vi "PCI8622模拟量采集.vi"() -> (0 "3通道":dbl, 1 "2通道":dbl, 2 "1通道":dbl, 3 "0通道":dbl)   [LabVIEW 2011]
panel:
  in  "超时时间(秒)":i32 min=0 max=3600
  in  "接地方式":i32(ring) items=["单端方式", "差分方式"]
  in  "触发灵敏窗(25nS)":i32=100 min=1 max=65535
  in  "分组间隔(uS)":i32=100 min=0 max=419430
  in  "采样频率(Hz)":i32=25000 min=0 max=250000
  in  "量程范围":i32(ring) items=["±10000mV", "±5000mV", "±2500mV", "0～10000mV", "0～5000mV"]
  in  "时钟输出":i32(ring) items=["禁止", "允许"]
  in  "时钟源选择":i32(ring) items=["内时钟", "外时钟"]
  in  "触发方向":i32(ring) items=["负向触发", "正向触发", "正负向触发"]
  in  "分组循环次数":i32=1 min=0 max=255
  in  "触发类型":i32(ring) items=["边沿触发", "脉冲触发"]
  in  "触发方式":i32(ring) items=["内触发", "后触发"]
  in  "程控增益":i32(ring) items=["1倍增益", "2倍增益", "5倍增益", "10倍增益"]
  in  "AD模式选择":i32(ring) items=["连续采样", "分组采样"]
  # "分组采样时\n每组频率"
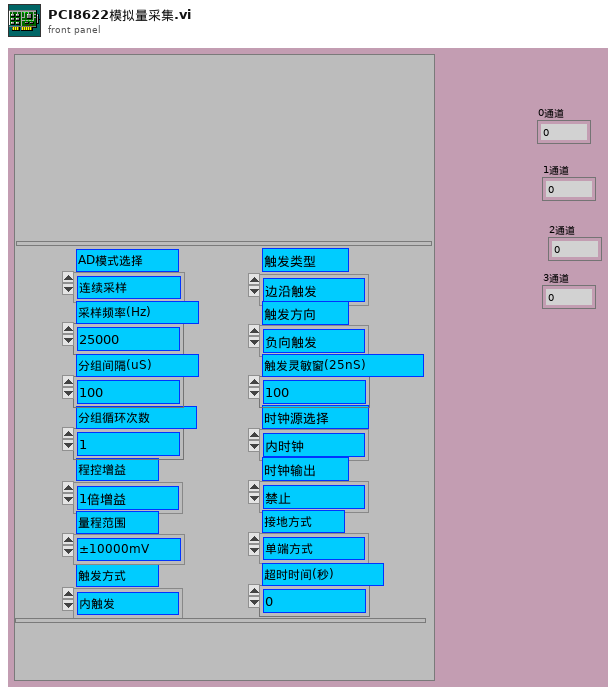
[diagram p1: front panel]
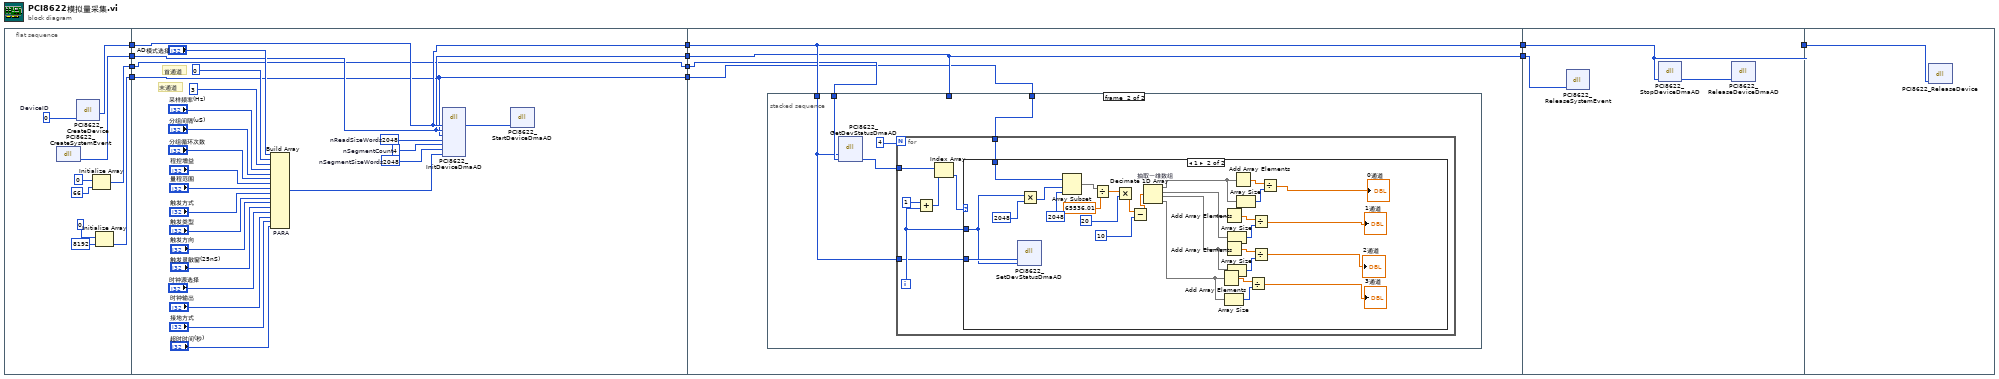
[diagram p0: block diagram]
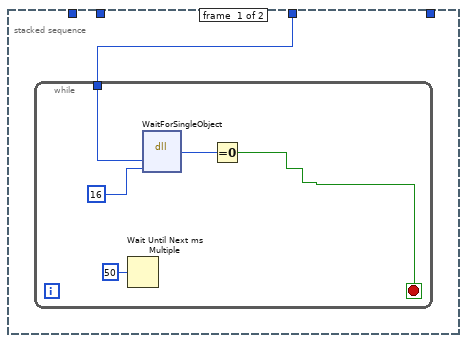
[diagram p2: hidden frame]
diagram:
  n1 = flat-sequence {
    tunnel: [w20] -> w11
    tunnel: [w18] -> w10
    tunnel: [w15] -> w9
    tunnel: [w12] -> w8
    tunnel: w11 -> [w29]
    tunnel: [w29] -> w7
    tunnel: w10 -> [w28]
    tunnel: [w28] -> w6
    tunnel: w9 -> [w21]
    tunnel: [w21] -> w5
    tunnel: w8 -> [w22]
    tunnel: [w22] -> w4
    tunnel: w7 -> [w49]
    tunnel: [w49] -> w3
    tunnel: w6 -> [w48]
    tunnel: [w48] -> w2
    tunnel: w5 -> [w47]
    tunnel: w4 -> [w46]
    tunnel: w3 -> [w98]
    tunnel: [w98] -> w1
    tunnel: w2 -> [w99]
    tunnel: w1 -> [w100]
    frame #0 {
      w19 = 0  # DeviceID
      n2 = dll-call lib="PCI8622" fn="PCI8622_CreateSystemEvent" label="CreateSystemEvent"() -> ("hEvent"=w18:i32)  [unwired: 3 in, 2 out]
      n3 = dll-call lib="PCI8622" fn="PCI8622_CreateDevice" label="CreateDevice"("DeviceID"=w19) -> (w20:i32)  [unwired: 4 in, 2 out]
      n4 = Initialize Array(0 ("element"), 66 ("dimension size")) -> (w15:i32[])
      n5 = Initialize Array(u16 0, 8192 ("dimension size")) -> (w12:u16[])
    }
    frame #1 {
      w24 = 2048  # nSegmentSizeWords
      w25 = 4  # nSegmentCount
      w27 = 2048  # nReadSizeWords
      # "末通道"
      # "首通道"
      n6 = Build Array "PARA"("AD模式选择", 0 ("首通道"), 3 ("末通道"), "采样频率(Hz)", "分组间隔(uS)", "分组循环次数", "程控增益", "量程范围", "触发方式", "触发类型", "触发方向", "触发灵敏窗(25nS)", "时钟源选择", "时钟输出", "接地方式", "超时时间(秒)") -> (w26:i32[])
      n7 = dll-call lib="PCI8622" fn="PCI8622_InitDeviceDmaAD" label="InitDeviceDmaAD"("hDevice"=w29, "hDmaEvent"=w28, "ADBuffer"=w22, "nReadSizeWords"=w27, "nSegmentCount"=w25, "nSegmentSizeWords"=w24, "pAPara"=w26) -> ("hDevice"=w23:i32)  [unwired: 10 in, 2 out]
      n8 = dll-call lib="PCI8622" fn="PCI8622_StartDeviceDmaAD" label="StartDeviceDmaAD"("hDevice"=w23) -> ()  [unwired: 5 in, 2 out]
    }
    frame #2 {
      n9 = stacked-sequence {
        tunnel: w48 -> [w50 _]
        tunnel: w49 -> [_ w56]
        tunnel: w47 -> [_ w60]
        tunnel: w46 -> [_ w57]
        frame #0 {
          n10 = while {
            tunnel: w50 -> [w52]
            stop <- w51 stop-if-true
            n11 = Wait Until Next ms Multiple(millisecond multiple=u32 50) -> ()  [unwired: 1 out]
            n12 = dll-call lib="kernel32" fn="WaitForSingleObject"("hEvent"=w52, "dwMilliseconds"=16) -> (w53:u32)  [unwired: 5 in, 2 out]
            n13 = Equal To 0?(x=w53) -> (x = 0?=w51:bool)
          }
        }
        frame #1 {
          n14 = dll-call lib="PCI8622" fn="PCI8622_GetDevStatusDmaAD" label="GetDevStatusDmaAD"("hDevice"=w56, "pDMAStatus"=w60) -> ("pDMAStatus"=w59:i32[])  [unwired: 5 in, 2 out]
          n15 = for {
            N: 4 -> [_]
            tunnel: w59 -> [w67]
            tunnel: w57 -> [w65]
            tunnel: w56 -> [w61]
            i -> [w63]
            n16 = Add(x=1, y=w63) -> (x+y=w62:i32)
            n17 = Index Array(array=w67, index=w62) -> (element=w66:i32)
            n18 = case shown="1" w66 {
              tunnel: w63 -> [_ w91]
              tunnel: w65 -> [_ w96]
              tunnel: w61 -> [_ w92]
              frame 0, Default {
              }
              frame 1 {
                n19 = dll-call lib="PCI8622" fn="PCI8622_SetDevStatusDmaAD" label="SetDevStatusDmaAD"("hDevice"=w92, "iClrBufferID"=w91) -> ()  [unwired: 6 in, 2 out]
                n20 = Multiply(x=w91, y=2048) -> (x*y=w93:i32)
                n21 = Array Subset(array=w96, index=w93, length=2048) -> (w89:u16[])
                n22 = Divide(x=w89, y=65536.01) -> (x/y=w90:dbl[])
                n23 = Multiply(x=w90, y=20) -> (x*y=w86:dbl[])
                n24 = Subtract(x=w86, y=10) -> (x-y=w84:dbl[])
                n25 = Decimate 1D Array "抽取一维数组"(w84) -> (w75:dbl[], w74:dbl[], w73:dbl[], w72:dbl[])
                n26 = Add Array Elements(numeric array=w72) -> (sum=w83:dbl)
                n27 = Array Size(array=w72) -> (size(s)=w76:i32)
                n28 = Add Array Elements(numeric array=w74) -> (sum=w79:dbl)
                n29 = Add Array Elements(numeric array=w73) -> (sum=w81:dbl)
                n30 = Array Size(array=w74) -> (size(s)=w80:i32)
                n31 = Array Size(array=w73) -> (size(s)=w82:i32)
                n32 = Add Array Elements(numeric array=w75) -> (sum=w77:dbl)
                n33 = Array Size(array=w75) -> (size(s)=w78:i32)
                n34 = Divide(x=w83, y=w76) -> (x/y=→"3通道":dbl)
                n35 = Divide(x=w79, y=w80) -> (x/y=→"1通道":dbl)
                n36 = Divide(x=w81, y=w82) -> (x/y=→"2通道":dbl)
                n37 = Divide(x=w77, y=w78) -> (x/y=→"0通道":dbl)
              }
            }
          }
        }
      }
    }
    frame #3 {
      n38 = dll-call lib="PCI8622" fn="PCI8622_ReleaseSystemEvent" label="ReleaseSystemEvent"("hEvent"=w99) -> ()  [unwired: 5 in, 2 out]
      n39 = dll-call lib="PCI8622" fn="PCI8622_StopDeviceDmaAD" label="StopDeviceDmaAD"("hDevice"=w98) -> ("hDevice"=w97:i32)  [unwired: 4 in, 2 out]
      n40 = dll-call lib="PCI8622" fn="PCI8622_ReleaseDeviceDmaAD" label="ReleaseDeviceDmaAD"("hDevice"=w97) -> ()  [unwired: 5 in, 2 out]
    }
    frame #4 {
      n41 = dll-call lib="PCI8622" fn="PCI8622_ReleaseDevice" label="ReleaseDevice"("hDevice"=w100) -> ()  [unwired: 5 in, 2 out]
    }
  }
